vi "ROI entry-Load and compare Z norm.vi"(8 "error in (no error)":errorcluster, 11 "Old ROI file path":path) -> (0 "error out":errorcluster, 1 "Both Zplane Pockels Values files exist":bool, 2 "All Z values in range":bool, 3 "Latest Zplane_Pockels_Values file data (header removed)":dbl[][](array[numeric]), 4 "Older [AOL Z (um)]":dbl[](array[numeric]), 5 "Latest [AOL Z (um)]":dbl[](array[numeric]), 6 "Older Zplane_Pockels_Values file data (header removed)":dbl[][](array[numeric]))   [LabVIEW 2020]
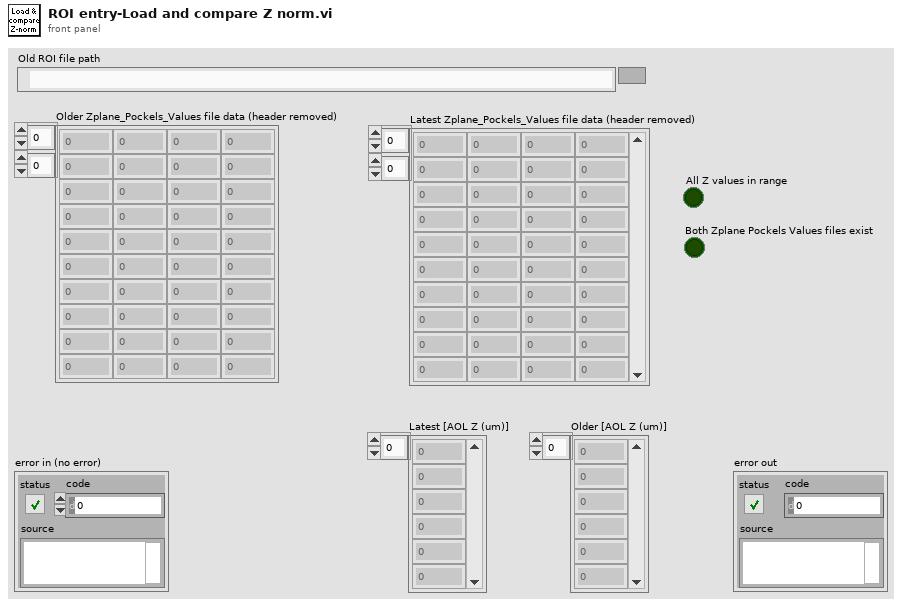
[diagram p1: front panel]
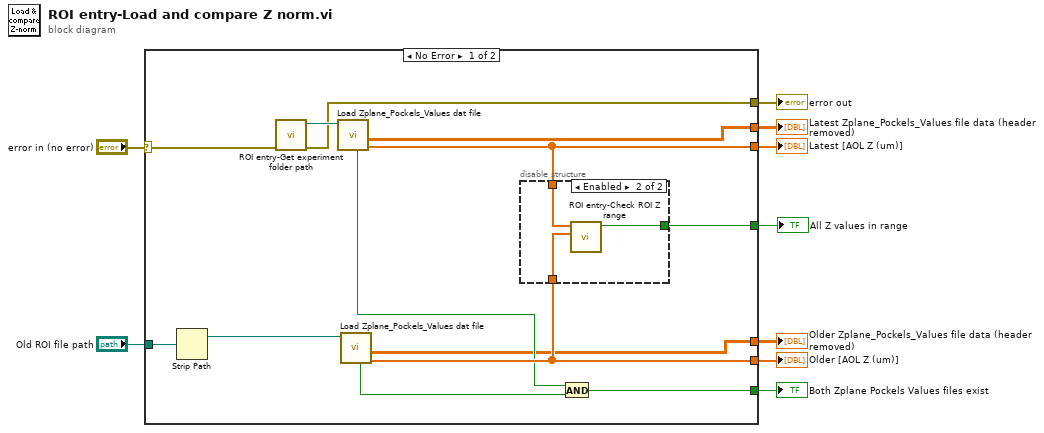
[diagram p0: block diagram]
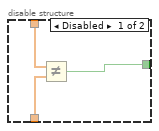
[diagram p2: hidden frame]
diagram:
  n1 = case shown="No Error" "error in (no error)" {
    selector: "error in (no error)" -> [w15 w29]
    tunnel: [w21 _] -> w9
    tunnel: [w20 _] -> w8
    tunnel: "Old ROI file path" -> [w18 _]
    tunnel: [w17 _] -> w6
    tunnel: [w16 _] -> w5
    tunnel: [w11 _] -> w4
    tunnel: [w14 w29] -> w2
    tunnel: [w10 _] -> w1
    frame No Error {
      n2 = Strip Path(path=w18) -> (stripped path=w19:path)  [unwired: 1 out]
      n3 = call "ROI entry-Get experiment folder path.vi"("error in (no error)"=w15) -> ("error out"=w14:errorcluster, "Experiment folder path"=w22:path)  [unwired: 9 in]
      n4 = call "Load Zplane_Pockels_Values dat file.vi"("Experiment data folder path"=w22) -> ("[AOL Z (um)]"=w17:dbl[], "Zplane_Pockels_Values file data (header removed)"=w21:dbl[][], "Zplane Pockels values file exists"=w12:bool)  [unwired: 5 in, 3 out]
      n5 = call "Load Zplane_Pockels_Values dat file.vi"("Experiment data folder path"=w19) -> ("[AOL Z (um)]"=w16:dbl[], "Zplane_Pockels_Values file data (header removed)"=w10:dbl[][], "Zplane Pockels values file exists"=w13:bool)  [unwired: 5 in, 3 out]
      n6 = disable-structure shown="Enabled" {
        disable-tunnel: [w25 w28] -> w20
        disable-tunnel: w17 -> [w24 w27]
        disable-tunnel: w16 -> [w23 w26]
        frame Disabled {
          n7 = Not Equal?(x=w24, y=w23) -> (x != y?=w25:bool)
        }
        frame Enabled {
          n8 = call "ROI entry-Check ROI Z range.vi"("[AOL Z  (um)] previous"=w26, "[AOL Z  (um)] Latest"=w27) -> ("All Z values in range ?"=w28:bool)  [unwired: 9 in]
        }
      }
      n9 = And(x=w12, y=w13) -> (x .and. y?=w11:bool)
    }
    frame Error {
    }
  }
  "Latest Zplane_Pockels_Values file data (header removed)" <- w9
  "All Z values in range" <- w8
  "Latest [AOL Z (um)]" <- w6
  "Older [AOL Z (um)]" <- w5
  "Both Zplane Pockels Values files exist" <- w4
  "error out" <- w2
  "Older Zplane_Pockels_Values file data (header removed)" <- w1
